vi "Tell.vi"(4 "Priority":bool, 10 "Msg":refnum<class "Msg.lvclass">, 11 "Notifier Transport in":refnum<class "Notifier Transport.lvclass">) -> (0 "Error out":errorcluster)   [LabVIEW 2025, in "jettl.lvlib" / "Transport.lvlib" / "Notifier.lvlib" / "Notifier Transport.lvclass"]
uses:
  Notifier Transport.lvclass
  Msg/Msg.lvclass
  Notifier Transport.lvclass/Notifier Transport.ctl
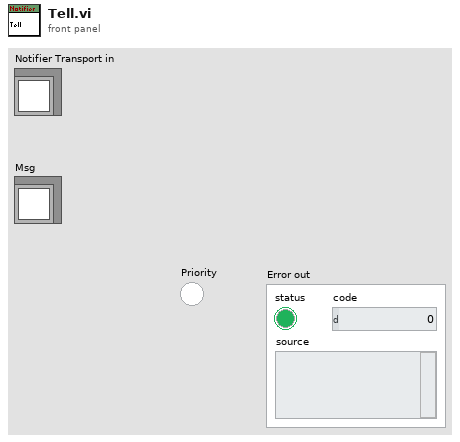
[diagram p1: front panel]
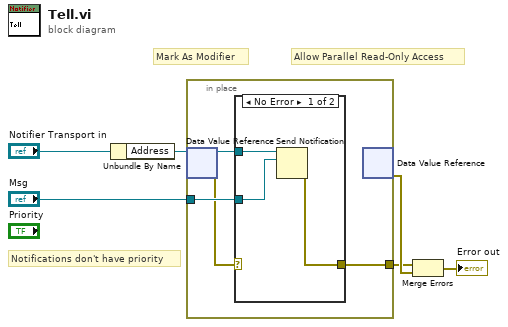
[diagram p0: block diagram]
diagram:
  # "Notifications don't have priority"
  # "Allow Parallel Read-Only Access"
  # "Mark As Modifier"
  n1 = Unbundle By Name("Notifier Transport in") -> ("Address"=w6:refnum<data-value>)
  n2 = in-place {
    in-place-border: [w10] -> w4
    in-place-border: "Msg" -> [w9]
    n3 = in-place-dvr #1(w6) -> (w8:refnum<notifier>, w7:errorcluster)
    n4 = case shown="No Error" w7 {
      selector: w7 -> [_ w14]
      tunnel: [w11 w14] -> w10
      tunnel: w9 -> [w12 _]
      tunnel: w8 -> [w13 _]
      frame No Error {
        n5 = Send Notification(notification=w12, notifier=w13) -> (error out=w11:errorcluster)  [unwired: 1 in, 1 out]
      }
      frame Error {
      }
    }
    n6 = in-place-dvr #1() -> (w5:errorcluster)  [unwired: 1 in, 1 out]
  }
  n7 = Merge Errors(w4, w5) -> (→"Error out":errorcluster)
